vi "Configure Composite Limit Test.vi"(0 "VISA resource name":refnum<visa-resource-name>, 1 "Enable Composite Limit Test (T: Enable)":bool=TRUE, 2 "Limit Test Feed Type (1: Current)":i32(ring)=1 items=["Math", "Current", "Resistance", "Charge", "Voltage"], 5 "Channel (1: Channel 1)":i32(ring)=1 items=["Channel 1"=1, "Channel 2"=2], 7 "Composite Limit Operation Type (1: Grading)":i32(ring)=1 items=["Sorting", "Grading"], 9 "Composite Limit Result Update Type (1: Immediate)":i32(ring)=1 items=["End", "Immediate"], 11 "error in (no error)":errorcluster, 12 "Composite Limit Fail Result Pattern (0)":i32, 13 "Composite Limit Pass Result Pattern (0)":i32) -> (4 "VISA resource name out":refnum<visa-resource-name>, 15 "error out":errorcluster)   [LabVIEW 2012, in "Keysight B2980 Series.lvlib"]
doc: "Configures the settings for composite limit test."
uses:
  Keysight B2980 Series.lvlib
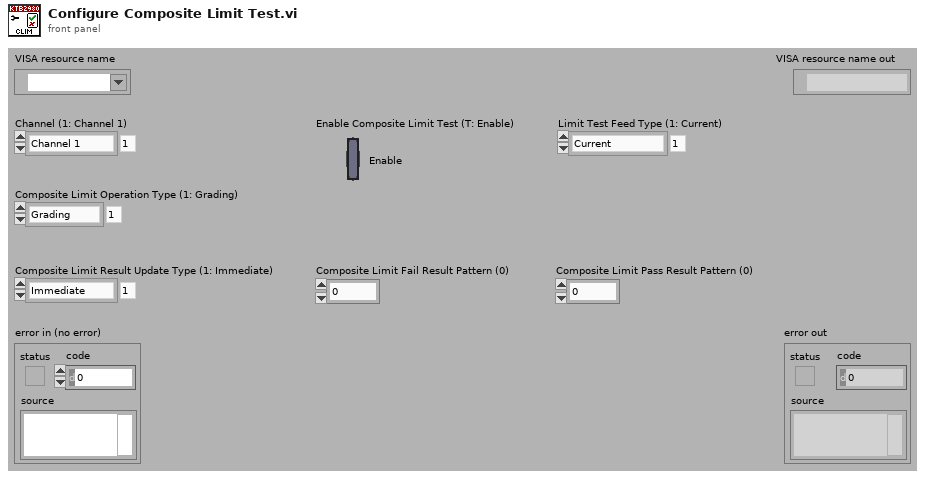
[diagram p1: front panel]
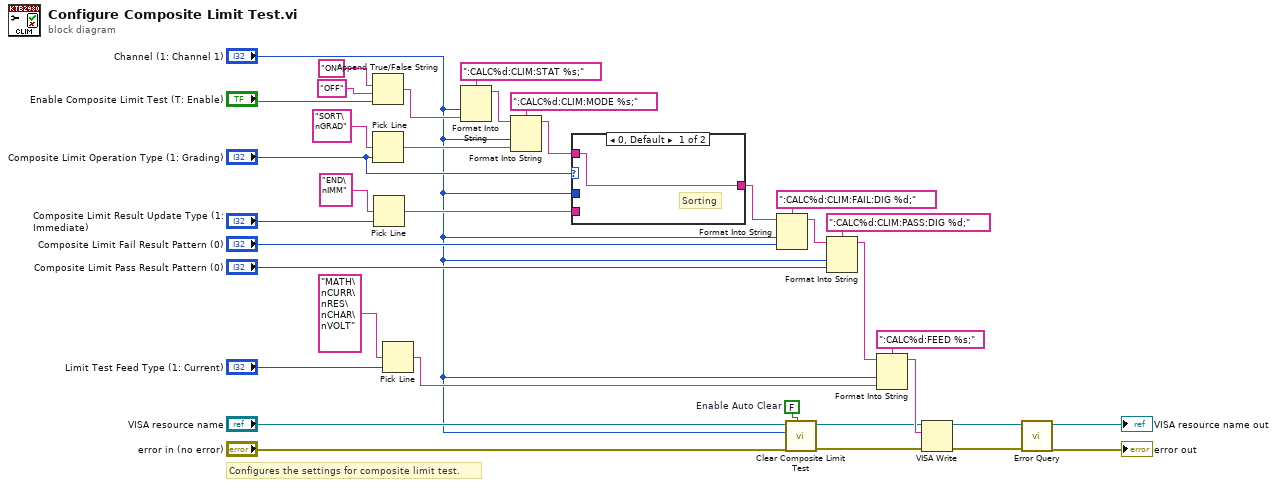
[diagram p0: block diagram]
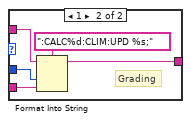
[diagram p2: hidden frame]
diagram:
  w2 = FALSE  # Enable Auto Clear
  # "Configures the settings for composite limit test."
  n1 = Append True/False String(1:"Enable Composite Limit Test (T: Enable)", 2:"OFF", 3:"ON") -> (0:w29:string)  [unwired: 1 out]
  n2 = Pick Line(multi-line string="SORT\nGRAD", line index="Composite Limit Operation Type (1: Grading)") -> (output string=w25:string)  [unwired: 1 out]
  n3 = Pick Line(multi-line string="END\nIMM", line index="Composite Limit Result Update Type (1: Immediate)") -> (output string=w34:string)  [unwired: 1 out]
  n4 = Pick Line(multi-line string="MATH\nCURR\nRES\nCHAR\nVOLT", line index="Limit Test Feed Type (1: Current)") -> (output string=w15:string)  [unwired: 1 out]
  n5 = Format Into String(format string=":CALC%d:CLIM:STAT %s;", "Channel (1: Channel 1)", w29) -> (resulting string=w27:string)  [unwired: 2 in, 1 out]
  n6 = Format Into String(format string=":CALC%d:CLIM:MODE %s;", initial string=w27, "Channel (1: Channel 1)", w25) -> (resulting string=w8:string)  [unwired: 1 in, 1 out]
  n7 = case shown="0, Default" "Composite Limit Operation Type (1: Grading)" {
    tunnel: w34 -> [_ w41]
    tunnel: "Channel (1: Channel 1)" -> [_ w40]
    tunnel: [w37 w39] -> w7
    tunnel: w8 -> [w37 w38]
    frame 0, Default {
      # "Sorting"
    }
    frame 1 {
      # "Grading"
      n8 = Format Into String(format string=":CALC%d:CLIM:UPD %s;", initial string=w38, w40, w41) -> (resulting string=w39:string)  [unwired: 1 in, 1 out]
    }
  }
  n9 = Format Into String(format string=":CALC%d:CLIM:FAIL:DIG %d;", initial string=w7, "Channel (1: Channel 1)", "Composite Limit Fail Result Pattern (0)") -> (resulting string=w22:string)  [unwired: 1 in, 1 out]
  n10 = call "Clear Composite Limit Test.vi"("Enable Auto Clear (T: Enable)"=w2, "error in (no error)"="error in (no error)", "Channel (1: Channel 1)"="Channel (1: Channel 1)", "VISA resource name"="VISA resource name") -> ("error out"=w3:errorcluster, "VISA resource name out"=w4:refnum<visa-resource-name>)  [unwired: 1 in, 5 out]
  n11 = Format Into String(format string=":CALC%d:CLIM:PASS:DIG %d;", initial string=w22, "Channel (1: Channel 1)", "Composite Limit Pass Result Pattern (0)") -> (resulting string=w17:string)  [unwired: 1 in, 1 out]
  n12 = Format Into String(format string=":CALC%d:FEED %s;", initial string=w17, "Channel (1: Channel 1)", w15) -> (resulting string=w14:string)  [unwired: 1 in, 1 out]
  n13 = VISA Write(VISA resource name=w4, write buffer=w14, error in (no error)=w3) -> (VISA resource name out=w13:refnum<visa-resource-name>, error out=w12:errorcluster)  [unwired: 1 out]
  n14 = call "Error Query.vi"("error in (no error)"=w12, "VISA resource name"=w13) -> ("error out"=→"error out":errorcluster, "VISA resource name out"=→"VISA resource name out":refnum<visa-resource-name>)  [unwired: 8 out]
